vi "update_rate_and_time.vi"(8 "error in (no error)":errorcluster) -> (0 "error out":errorcluster, 2 "time (ms)":u32, 3 "rate (Hz)":dbl)   [LabVIEW 2016]
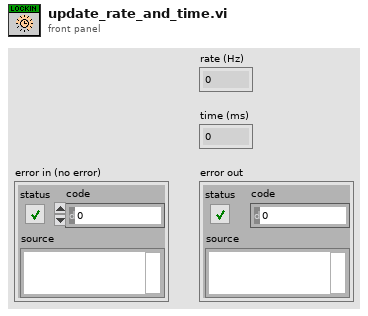
[diagram p1: front panel]
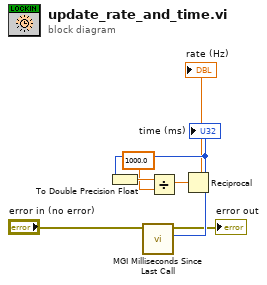
[diagram p0: block diagram]
diagram:
  n1 = call <userlib>:"MGI Milliseconds Since Last Call.vi"("Error In"="error in (no error)") -> ("ms"=w7:u32, "Error Out"=→"error out":errorcluster)  [unwired: 5 in]
  "time (ms)" <- w7
  n2 = To Double Precision Float(number=w7) -> (double precision float=w3:dbl)
  n3 = Divide(x=w3, y=1000.0 ("x")) -> (x/y=w1:dbl)
  n4 = Reciprocal(x=w1) -> (1/x=→"rate (Hz)":dbl)
